vi "DifferentPrototype.vi"(6 "String In":string, 7 "Numeric In":dbl format="%.2f", 8 "String To Append":string, 9 "Number To Multiply":dbl format="%.2f") -> (2 "String Out":string, 3 "Numeric Out":dbl format="%.2f")   [LabVIEW 2013]
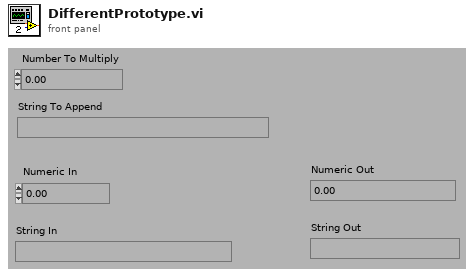
[diagram p1: front panel]
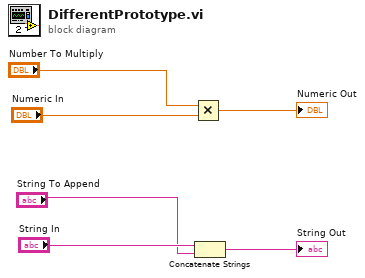
[diagram p0: block diagram]
diagram:
  n1 = Multiply(x="Number To Multiply", y="Numeric In") -> (x*y=→"Numeric Out":dbl)
  n2 = Concatenate Strings("String In", "String To Append") -> (→"String Out":string)
